vi "SUM OF N NUMBERS.vi"() -> ()   [LabVIEW 2017]
panel:
  out "Numeric Indicator 2":dbl
  out "Array":dbl[](array[numeric])
  out "Numeric Indicator":dbl
  # "SUM OF N NUMBERS"
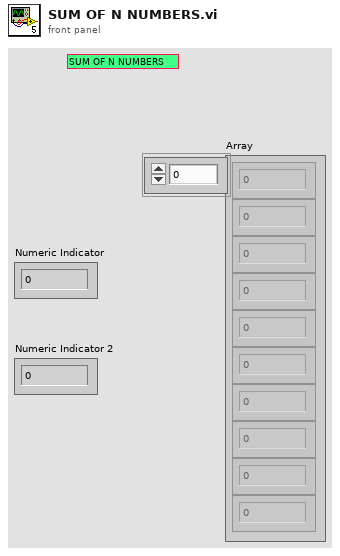
[diagram p1: front panel]
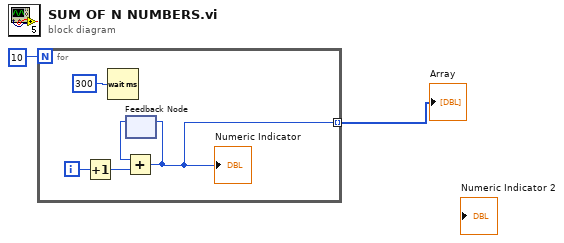
[diagram p0: block diagram]
diagram:
  n1 = for {
    N: 10 -> [_]
    tunnel: [w3] -> w1 mode=indexing
    i -> [w6]
    n2 = Increment(x=w6) -> (x+1=w7:i32)
    n3 = Wait (ms)(milliseconds to wait=u32 300) -> ()  [unwired: 1 out]
    n4 = feedback #1() -> (w5:i32)  [unwired: 1 in]
    n5 = Add(x=w5, y=w7) -> (x+y=w3:i32)
    "Numeric Indicator" <- w3
    n6 = feedback-in #1(w3) -> ()
  }
  "Array" <- w1
